vi "Power.vi"(5 "Negative Power":dbl, 7 "Positive Power":dbl, 9 "Negative":bool, 10 "Positive":bool) -> (2 "Output":dbl)   [LabVIEW 2020, in "TitanLib.lvlib"]
uses:
  TitanLib.lvlib
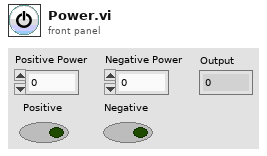
[diagram p1: front panel]
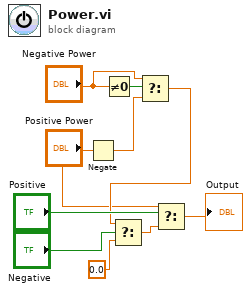
[diagram p0: block diagram]
diagram:
  n1 = Negate(x="Positive Power") -> (-x=w2:dbl)
  n2 = Not Equal To 0?(x="Negative Power") -> (x != 0?=w5:bool)
  n3 = Select(t="Negative Power", s=w5, f=w2) -> (s? t:f=w3:dbl)
  n4 = Select(t=w3, s="Negative", f=0.0) -> (s? t:f=w10:dbl)
  n5 = Select(t="Positive Power", s="Positive", f=w10) -> (s? t:f=→"Output":dbl)
